vi "Autophase.vi"(8 "error in (no error)":errorcluster, 9 "Boolean":bool, 10 "Results":T1 {"Results (Dictionary)"."value" format="%#_6p"}, 11 "Instrument.DAQ in":refnum<class "Instrument.DAQ.lvclass">) -> (0 "error out":errorcluster, 3 "Instrument.DAQ out":refnum<class "Instrument.DAQ.lvclass">)   [LabVIEW 2019, in "Instrument.Lockin.lvlib" / "Instrument.DAQ.lvclass"]
uses:
  Instrument.DAQ.lvclass
  Typedefs/Results--Cluster.ctl
  Instrument.DAQ.lvclass/Instrument.DAQ.ctl
  Instrument.Lockin/Typedefs/Results Type--Enum.ctl
  <vilib>/addons/control/pid/pid.llb/PID (DBL Array).vi
  Instrument.Lockin/Instrument.Lockin.lvclass
  <vilib>/addons/control/pid/NI_PID_pid.lvlib
  <vilib>/addons/control/pid/pid.llb/PID Control Input Filter (DBL).vi
panel:
  out "output":dbl[](array[numeric]) format="%.2f"
  in  "D":dbl=0.019999999999999997 format="%.3f"
  in  "I":dbl=0.6 format="%.3f"
  in  "P":dbl=0.5 format="%.2f"
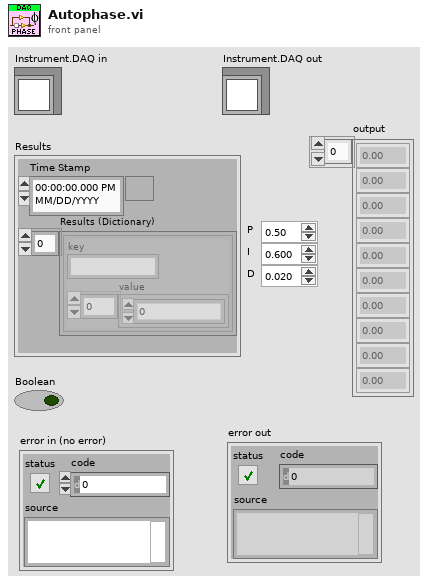
[diagram p1: front panel]
types:
  T1 = typedef "Instrument.Lockin.lvlib/Instrument.DAQ.lvclass/Results--Cluster.ctl" = cluster{"Time Stamp":timestamp, "Results (Dictionary)":cluster{"key":string, "value":dbl[]}[]}
  T2 = cluster{"proportional gain (Kc)":dbl, "integral time (Ti, min)":dbl, "derivative time (Td, min)":dbl}
  T3 = typedef "Instrument.Lockin.lvlib/Instrument.Lockin.lvclass/Results Type--Enum.ctl" = enum16{"X", "Y", "R", "Theta", "Mean"}
  T4 = typedef "Instrument.Lockin.lvlib/Instrument.DAQ.lvclass/AO.Channel--Cluster--Array.ctl" = T5[]
  T5 = typedef "Instrument.Lockin.lvlib/Instrument.DAQ.lvclass/AO.Channel--Cluster.ctl" = cluster{"Enable?":bool, "Channel":i32, "Amplitude":dbl, "Offset":dbl, "Frequency":dbl, "Phase":dbl, "Function":T6, "Sweeping?":bool, "Limit AC":bool, "Limit DC?":bool, "Duty Cycle":bool}
  T6 = typedef "Instrument.Lockin.lvlib/Instrument.DAQ.lvclass/AO.Channel.Function--Enum.ctl" = enum16{"sine", "square", "triangle", "saw"}
  T7 = cluster{"proportional gain (Kc)":dbl, "integral time (Ti, min)":dbl, "derivative time (Td, min)":dbl}[]
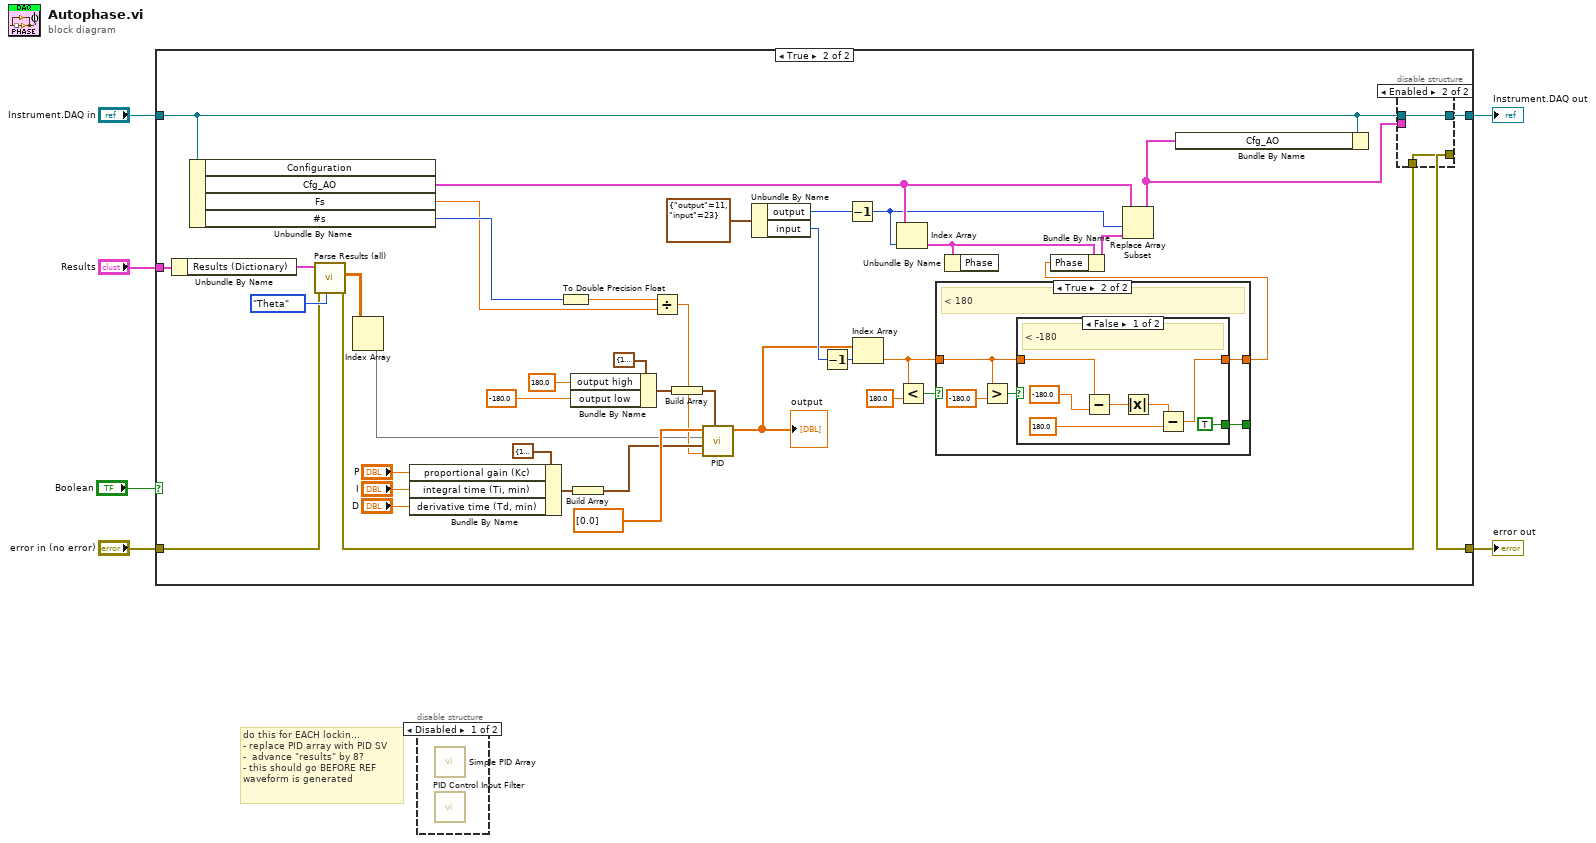
[diagram p0: block diagram]
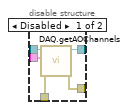
[diagram p3: hidden frame]
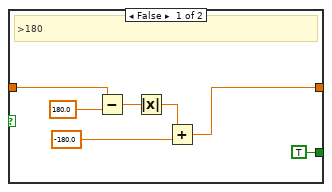
[diagram p4: hidden frame]
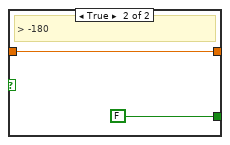
[diagram p5: hidden frame]
diagram:
  # "do this for EACH lockin...\n- replace PID array with PID SV\n-  advance \"results\" by 8?\n- this should go BEFORE REF\nwaveform is generated"
  n1 = case shown="True" "Boolean" {
    tunnel: "Instrument.DAQ in" -> [w8 w10]
    tunnel: "Results" -> [_ w48]
    tunnel: "error in (no error)" -> [w7 w12]
    tunnel: [w8 w47] -> w3
    tunnel: [w7 w13] -> w2
    frame False {
    }
    frame True {
      n2 = Unbundle By Name(w48) -> ("Results (Dictionary)"=w46:cluster{"key":string, "value":dbl[]}[])
      n3 = Unbundle By Name(w10) -> ("Cfg_AO"=w31:T4, "Fs"=w21:dbl, "#s"=w22:i32)  [unwired: 1 out]
      n4 = call "Parse Results (all).vi"("Type"=Results_Type--Enum."Theta", "error in (no error)"=w12, "Results (Dictionary)"=w46) -> ("error out"=w44:errorcluster, "Data"=w11:dbl[][])  [unwired: 5 in, 2 out]
      n5 = Index Array(array=w11) -> (element=w9:dbl[])  [unwired: 2 in]
      n6 = Bundle By Name(cluster=T2 {"proportional gain (Kc)"=1.0, "integral time (Ti, min)"=0.01, "derivative time (Td, min)"=0.0} ("PID gains"), "proportional gain (Kc)"="P", "integral time (Ti, min)"="I", "derivative time (Td, min)"="D") -> (w37:T2)
      n7 = To Double Precision Float(number=w22) -> (double precision float=w14:dbl)
      n8 = Bundle By Name(cluster=cluster{"output high":dbl, "output low":dbl} {"output high"=100.0, "output low"=-100.0} ("output range"), "output high"=180.0, "output low"=-180.0) -> (w38:cluster{"output high":dbl, "output low":dbl})
      n9 = Build Array(w37) -> (w33:T7)
      n10 = Divide(x=w14, y=w21) -> (x/y=w20:dbl)
      n11 = Build Array(w38) -> (w29:cluster{"output high":dbl, "output low":dbl}[])
      n12 = call-poly <vilib>:"PID.vi"("output range"=w29, "dt (s)"=w20, "PID gains"=w33, "process variable"=w9, "setpoint"=dbl[] [0.0]) -> ("output"=w19:dbl[])  [unwired: 5 in, 1 out]
      "output" <- w19
      n13 = Unbundle By Name(cluster{"output":i32, "input":i32} {"output"=11, "input"=23}) -> ("output"=w27:i32, "input"=w26:i32)
      n14 = Decrement(x=w26) -> (x-1=w25:i32)
      n15 = Decrement(x=w27) -> (x-1=w24:i32)
      n16 = Index Array(array=w19, index=w25) -> (element=w16:dbl)
      n17 = Index Array(array=w31, index=w24) -> (element=w32:T5)
      n18 = Less?(x=w16, y=180.0) -> (x < y?=w17:bool)
      n19 = case shown="True" w17 {
        tunnel: w16 -> [w58 w64]
        tunnel: [w57 w65] -> w15
        tunnel: [TRUE w63] -> _
        frame False {
          # ">180"
          n20 = Subtract(x=w58, y=180.0) -> (x-y=w61:dbl)
          n21 = Absolute Value(x=w61) -> (abs(x)=w60:dbl)
          n22 = Add(x=w60, y=-180.0) -> (x+y=w57:dbl)
        }
        frame True {
          # "< 180"
          n23 = Greater?(x=w64, y=-180.0) -> (0:w67:bool)
          n24 = case shown="False" w67 {
            tunnel: [w69 w76] -> w65
            tunnel: w64 -> [w70 w76]
            tunnel: [TRUE FALSE] -> w63
            frame False {
              # "< -180"
              n25 = Subtract(x=w70, y=-180.0) -> (x-y=w73:dbl)
              n26 = Absolute Value(x=w73) -> (abs(x)=w72:dbl)
              n27 = Subtract(x=w72, y=180.0) -> (x-y=w69:dbl)
            }
            frame True {
              # "> -180"
            }
          }
        }
      }
      n28 = Unbundle By Name(w32) -> ()  [unwired: 1 out]
      n29 = Bundle By Name(cluster=w32, "Phase"=w15) -> (w30:T5)
      n30 = Replace Array Subset(array=w31, new element=w30, index=w24) -> (w23:T4)
      n31 = Bundle By Name(cluster=w10, "Cfg_AO"=w23) -> ()  [unwired: 1 out]
      n32 = disable-structure shown="Enabled" {
        disable-tunnel: [w53 w55] -> w47
        disable-tunnel: w10 -> [w52 w55]
        disable-tunnel: w44 -> [w51 w54]
        disable-tunnel: w23 -> [w50 _]
        disable-tunnel: [w49 w54] -> w13
        frame Disabled {
          n33 = call "DAQ.getAOChannels.vi"("error in (no error)"=w51, "Channels: AO"=w50, "Instrument.DAQ"=w52) -> ("error out"=w49:errorcluster, "Instrument.DAQ out"=w53:refnum<class "Instrument.DAQ.lvclass">)  [unwired: 7 in]
        }
        frame Enabled {
        }
      }
    }
  }
  "Instrument.DAQ out" <- w3
  "error out" <- w2
  n34 = disable-structure shown="Disabled" {
    frame Disabled {
      n35 = call "Simple PID Array.vi"() -> ()  [unwired: 11 in, 1 out]
      n36 = call-poly <vilib>:"PID Control Input Filter.vi"() -> ()  [unwired: 5 in, 1 out]
    }
    frame Enabled {
    }
  }
